vi "Run Action.vi"(8 "error in (no error)":errorcluster, 11 "GPackCLI in":refnum<class "GPackCLI.lvclass">) -> (0 "error out":errorcluster, 3 "GPackCLI out":refnum<class "GPackCLI.lvclass">)   [LabVIEW 2020, in "GPackTools.lvlib" / "GPackCLI.lvclass"]
uses:
  GPackCLI.lvclass
  GPackCLI.lvclass/GPackCLI.ctl
  CLILogger/CLILogger.lvclass
  C:/dev/lv20CE/relink/lv-gpack/GPack/Logger/Logger.lvclass
  CLIAction/CLIAction.lvclass
  GPack/Logger/Logger.lvclass
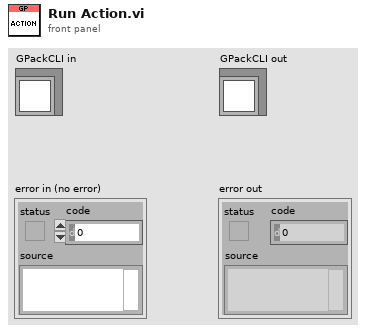
[diagram p1: front panel]
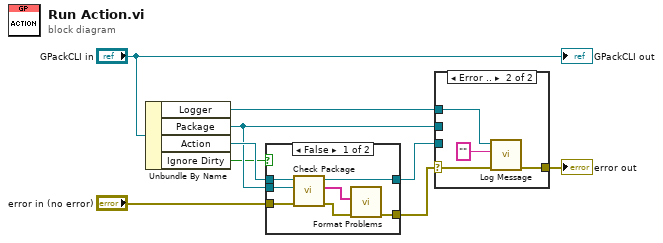
[diagram p0: block diagram]
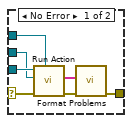
[diagram p3: hidden frame]
diagram:
  n1 = Unbundle By Name("GPackCLI in") -> ("Logger"=w2:refnum<class "CLILogger.lvclass">, "Package"=w3:refnum<class "PackageAbstract.lvclass">, "Action"=w6:refnum<class "CLIAction.lvclass">, "Ignore Dirty"=w1:bool)
  n2 = case shown="False" w1 {
    tunnel: "error in (no error)" -> [w16 w17]
    tunnel: w6 -> [w15 w18]
    tunnel: [w14 w18] -> w5
    tunnel: [w11 w17] -> w4
    tunnel: w3 -> [w10 _]
    frame False {
      n3 = call-dynamic "Check Package.vi"("error in (no error)"=w16, "Package"=w10, "CLIAction in"=w15) -> ("error out"=w12:errorcluster, "Problems"=w13:string[], "CLIAction out"=w14:refnum<class "CLIAction.lvclass">)  [unwired: 6 in]
      n4 = call "Format Problems.vi"("error in (no error)"=w12, "Problems"=w13) -> ("error out"=w11:errorcluster)  [unwired: 9 in]
    }
    frame True {
    }
  }
  n5 = case shown="Error .." w4 {
    selector: w4 -> [w21 w29]
    tunnel: [w24 w28] -> w7
    tunnel: w5 -> [w22 _]
    tunnel: w3 -> [w20 _]
    tunnel: w2 -> [w19 w27]
    frame No Error {
      n6 = call-dynamic "Run Action.vi"("Logger"=w19, "error in (no error)"=w21, "Package"=w20, "CLIAction in"=w22) -> ("error out"=w25:errorcluster, "Problems"=w23:string[])  [unwired: 5 in, 1 out]
      n7 = call "Format Problems.vi"("error in (no error)"=w25, "Problems"=w23) -> ("error out"=w24:errorcluster)  [unwired: 9 in]
    }
    frame Error {
      n8 = call "Log Message.vi"("error in (no error)"=w29, "Message"="", "Logger in"=w27) -> ("error out"=w28:errorcluster)  [unwired: 7 in, 1 out]
    }
  }
  "error out" <- w7
  "GPackCLI out" <- "GPackCLI in"
